vi "calculate_scrollbar_doc_max.vi"(5 "visible_columns":i32, 7 "visible_rows":i32, 8 "error in (no error)":errorcluster, 10 "data_columns":i32, 11 "data_rows":i32) -> (0 "error out":errorcluster, 4 "horizontal":dbl, 6 "vertical":dbl)   [LabVIEW 2015, in "lv-pagination.lvlib"]
doc: "This VI will take the values of the visible rows/columns and the amount of data rows/columns and computer the document max for vertical and horizontal scrollbars. This is 100% dependent on the accuracy of calculating the visible rows."
uses:
  lv-pagination.lvlib
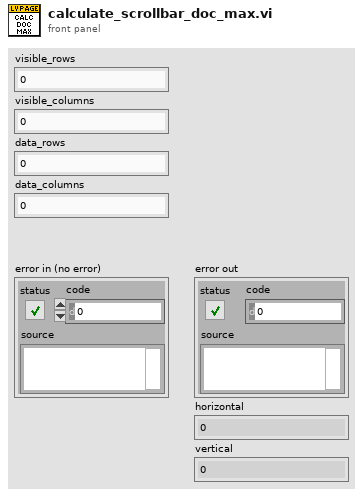
[diagram p1: front panel]
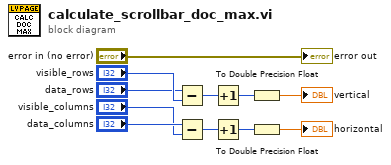
[diagram p0: block diagram]
diagram:
  n1 = Subtract(x="data_rows", y="visible_rows") -> (x-y=w9:i32)
  n2 = Subtract(x="data_columns", y="visible_columns") -> (x-y=w2:i32)
  n3 = Increment(x=w9) -> (x+1=w3:i32)
  n4 = Increment(x=w2) -> (x+1=w1:i32)
  n5 = To Double Precision Float(number=w3) -> (double precision float=→"vertical":dbl)
  n6 = To Double Precision Float(number=w1) -> (double precision float=→"horizontal":dbl)
  "error out" <- "error in (no error)"
